vi "IMAQdx Read Register2.vi"(8 "error in":errorcluster, 10 "Offset":u64=4042262528 format="%.0x", 11 "Session In":T1) -> (0 "error out":errorcluster, 1 "Value":u32 format="%.0x", 3 "Session Out":T1)   [LabVIEW 2020, in "NI_Vision_Acquisition_Software.lvlib"]
doc: "Accesses registers on the camera and reads a 32-bit value from the camera. Data is byte-swapped for little endian alignment after transfer."
uses:
  NI_Vision_Acquisition_Software.lvlib
  IMAQdx.ctl
  niimaqdx.dll
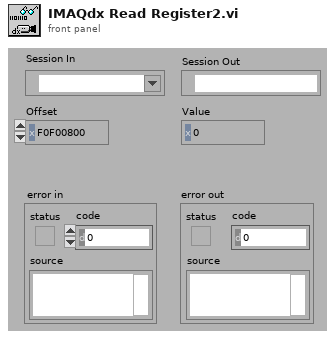
[diagram p1: front panel]
types:
  T1 = typedef "IMAQdx.ctl" = refnum<k21>
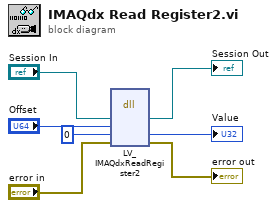
[diagram p0: block diagram]
diagram:
  n1 = dll-call lib="niimaqdx.dll" fn="LV_IMAQdxReadRegister2"("refNum"="Session In", "offset"="Offset", "value"=u32 0, "err"="error in") -> ("refNum"=→"Session Out":T1, "value"=→"Value":u32, "err"=→"error out":errorcluster)  [unwired: 5 in, 2 out]
